vi "GetAttributeViInt32_SS-DMod_ListSeq_RF.vi"(8 "error in (no error)":errorcluster {"code" format="%.0x"}, 9 "AttributeID":u32(ring)=1150908 items=["SS_DIGITALMODULATION_ARB_ALC_HOLD "=1150908, "SS_DIGITALMODULATION_ARB_CONTINUOUS_TRIGGER_TYPE "=1150883, "SS_DIGITALMODULATION_ARB_EXTERNAL_TRIGGER_SLOPE "=1150885, "SS_DIGITALMODULATION_ARB_RE_TRIGGER_MODE "=1150888, "SS_DIGITALMODULATION_ARB_RF_BLANKING "=1150909, "SS_DIGITALMODULATION_ARB_RMS_CALCULATION_MODE"=1150892, "SS_DIGITALMODULATION_ARB_SEGMENT_ADVANCE_TRIGGER_TYPE "=1150884, "SS_DIGITALMODULATION_ARB_TRIGGER_SOURCE "=1150881, "SS_DIGITALMODULATION_ARB_TRIGGER_TYPE "=1150882, "SS_LISTSEQUENCER_REPEATITION_MODE "=1150904, "SS_LISTSEQUENCER_SETUP_NUMBER_OF_STEPS "=1150905, "SS_LISTSEQUENCER_SETUP_TRIGGER_TYPE "=1150906, "SS_RFGENERATOR_MODULATION_ANALOG_FORMAT"=1150935, "SS_RFGENERATOR_MODULATION_ANALOG_WAVEFORM_TYPE "=1150936, "SS_RFGENERATOR_MODULATION_TYPE "=1150941, "SS_RFGENERATOR_RADIO_BAND "=1150911, "SS_RFGENERATOR_RADIO_CHANNEL_NUMBER "=1150910], 10 "RepCapIdentifier":string, 11 "instrument handle":refnum<k15>) -> (0 "error out":errorcluster {"code" format="%.0x"}, 2 "AttributeValue":i32, 3 "instrument handle out":refnum<k15>)   [LabVIEW 2009, in "Keysight XSAn.lvlib"]
doc: "Gets an Int32 attribute from the instrument driver.\nThe following Attributes are supported:\n\nSS_DIGITALMODULATION_ARB_ALC_HOLD \nSS_DIGITALMODULATION_ARB_CONTINUOUS_TRIGGER_TYPE \nSS_DIGITALMODULATION_ARB_EXTERNAL_TRIGGER_SLOPE \nSS_DIGITALMODULATION_ARB_RE_TRIGGER_MODE \nSS_DIGITALMODULATION_ARB_RF_BLANKING \nSS_DIGITALMODULATION_ARB_RMS_CALCULATION_MODE\nSS_DIGITALMODULATION_ARB_SEGMENT_ADVANCE_TRIGGER_TYPE \nSS_DIGITALMODULATION_ARB_TRIGGER_SOURCE \nSS_DIGITALMODULATION_ARB_TRIGGER_TYPE \nSS_LISTSEQUENCER_REPEATITION_MODE \nSS_LISTSEQUENCER_SETUP_NUMBER_OF_STEPS \nSS_LISTSEQUENCER_SETUP_TRIGGER_TYPE \nSS_RFGENERATOR_MODULATION_ANALOG_FORMAT\nSS_RFGENERATOR_MODULATION_ANALOG_WAVEFORM_TYPE \nSS_RFGENERATOR_MODULATION_TYPE \nSS_RFGENERATOR_RADIO_BAND \nSS_RFGENERATOR_RADIO_CHANNEL_NUMBER"
uses:
  <instrlib>/Keysight XSAn/Keysight XSAn.lvlib
  AgXSAn.dll
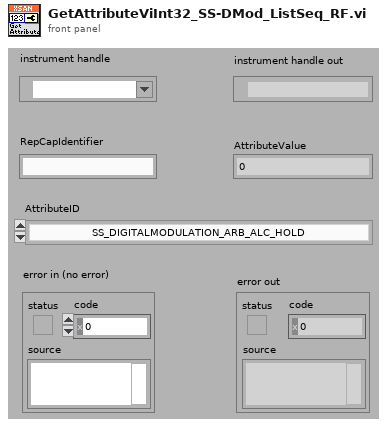
[diagram p1: front panel]
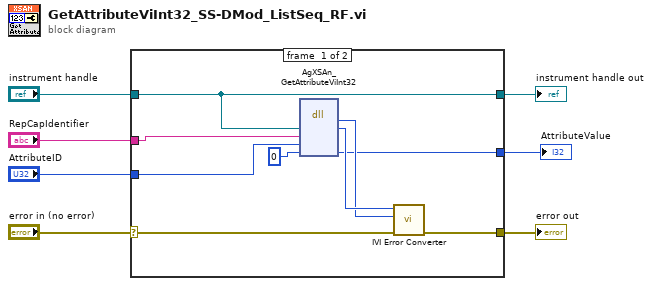
[diagram p0: block diagram]
diagram:
  n1 = case shown="No Error" "error in (no error)" {
    selector: "error in (no error)" -> [w14 w18]
    tunnel: [w13 w18] -> w7
    tunnel: "instrument handle" -> [w8 w17]
    tunnel: "RepCapIdentifier" -> [w12 _]
    tunnel: "AttributeID" -> [w11 _]
    tunnel: [w9 _] -> w2
    tunnel: [w8 w17] -> w1
    frame #0 {
      n2 = dll-call lib="AgXSAn**.dll" fn="AgXSAn_GetAttributeViInt32"("Vi"=w8, "RepCapIdentifier"=w12, "AttributeID"=w11, "AttributeValue"=0) -> ("return type"=w15:i32, "Vi"=w16:u32, "AttributeValue"=w9:i32)  [unwired: 5 in, 2 out]
      n3 = call <instrlib>:"IVI Error Converter.vi"("error in (no error)"=w14, "IVI error code (0)"=w15, "instrument handle"=w16) -> ("error out"=w13:errorcluster)  [unwired: 7 in, 1 out]
    }
    frame #1 {
    }
  }
  "error out" <- w7
  "instrument handle out" <- w1
  "AttributeValue" <- w2
